vi "Interpret_LiDAR_Return_Data.vi"(11 "Remaining Data in":u8[](array[numeric])) -> (2 "Return Data out":T1 {"Reflectance" format="%.6f %"; "Range" format="%.4f M"; "Existence Probability" format="%.4f %"}, 3 "Remaining Data out":u8[](array[numeric]))   [LabVIEW 2018, in "LiDAR.lvlib" / "LiDAR.lvclass"]
uses:
  LiDAR.lvclass
  Controls/cls_Point_Cloud_Return_Data.ctl
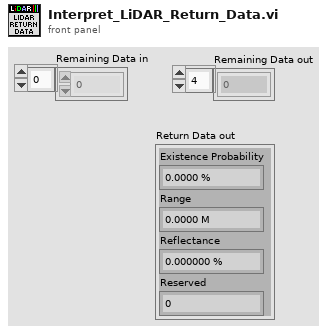
[diagram p1: front panel]
types:
  T1 = typedef "LiDAR.lvlib/LiDAR.lvclass/cls_Point_Cloud_Return_Data.ctl" = cluster{"Existence Probability":dbl, "Range":dbl, "Reflectance":dbl, "Reserved":u16}
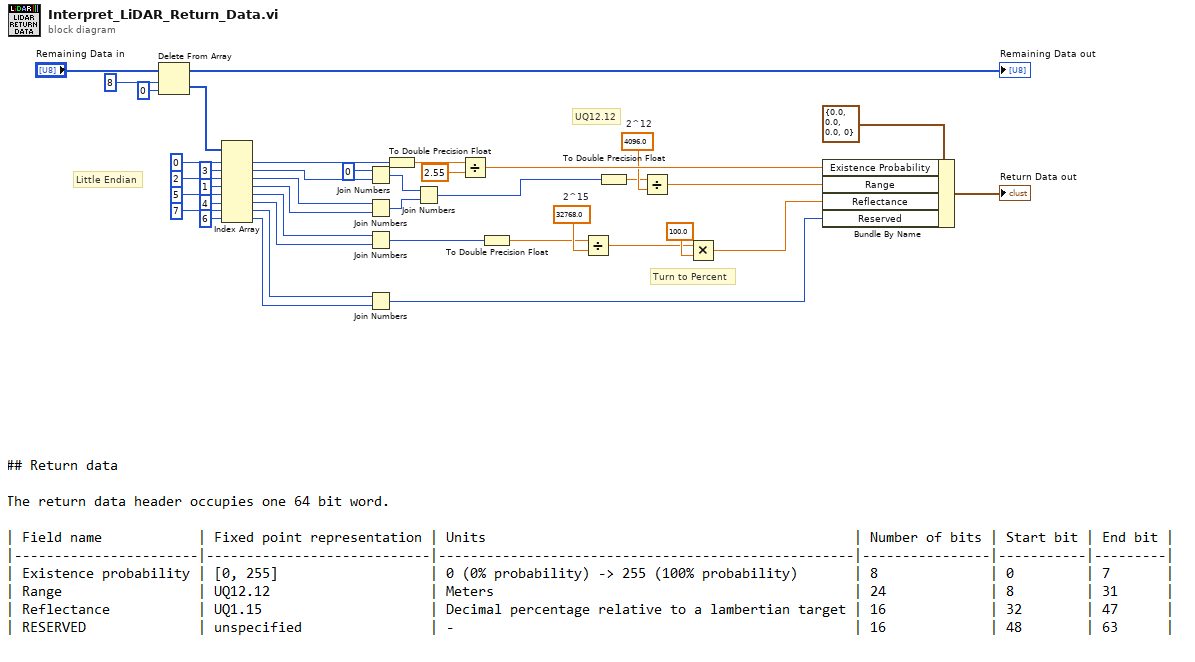
[diagram p0: block diagram]
diagram:
  w21 = 32768.0  # 2^15
  w22 = 4096.0  # 2^12
  # "Turn to Percent"
  # "UQ12.12"
  # "Little Endian"
  n1 = Delete From Array(array="Remaining Data in", length=8, index=0) -> (deleted portion=w38:u8[], array with subset deleted=→"Remaining Data out":u8[])
  n2 = Index Array(array=w38, index #1=0 ("index"), index #2=3 ("index"), index #3=2 ("index"), index #4=1 ("index"), index #5=5 ("index"), index #6=4 ("index"), index #7=7 ("index"), index #8=6 ("index")) -> (element #1=w25:u8, element #2=w18:u8, element #3=w14:u8, element #4=w13:u8, element #5=w34:u8, element #6=w33:u8, element #7=w32:u8, element #8=w31:u8)
  n3 = Join Numbers(hi=u8 0 ("lo"), lo=w18) -> ((hi.lo)=w36:u16)
  n4 = Join Numbers(hi=w14, lo=w13) -> ((hi.lo)=w35:u16)
  n5 = Join Numbers(hi=w34, lo=w33) -> ((hi.lo)=w3:u16)
  n6 = Join Numbers(hi=w32, lo=w31) -> ((hi.lo)=w30:u16)
  n7 = To Double Precision Float(number=w25) -> (double precision float=w6:dbl)
  n8 = Join Numbers(hi=w36, lo=w35) -> ((hi.lo)=w5:u32)
  n9 = Divide(x=w6, y=2.55) -> (x/y=w23:dbl)
  n10 = To Double Precision Float(number=w3) -> (double precision float=w2:dbl)
  n11 = Divide(x=w2, y=w21) -> (x/y=w1:dbl)
  n12 = To Double Precision Float(number=w5) -> (double precision float=w9:dbl)
  n13 = Divide(x=w9, y=w22) -> (x/y=w4:dbl)
  n14 = Multiply(x=w1, y=100.0) -> (x*y=w8:dbl)
  n15 = Bundle By Name(cluster=T1 {"Existence Probability"=0.0, "Range"=0.0, "Reflectance"=0.0, "Reserved"=0} ("Point Cloud Return Data"), "Existence Probability"=w23, "Range"=w4, "Reflectance"=w8, "Reserved"=w30) -> (→"Return Data out":T1)
